vi "HelloWorld.vi"() -> ()   [LabVIEW 2018]
panel:
  out "error out":errorcluster
  in  "Name":string="World"
  out "response":string
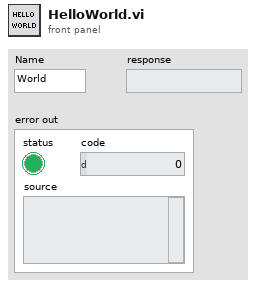
[diagram p1: front panel]
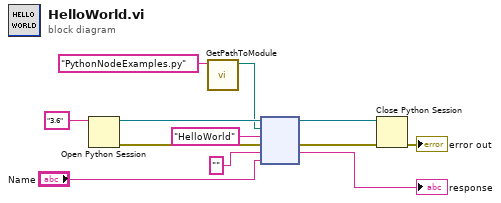
[diagram p0: block diagram]
diagram:
  n1 = Open Python Session(python version="3.6" ("Python version")) -> (session out=w12:refnum<k35>, error out=w4:errorcluster)  [unwired: 2 in]
  n2 = call "GetPathToModule.vi"("module name"="PythonNodeExamples.py") -> ("path to module"=w5:path)  [unwired: 10 in]
  n3 = node(w12, w5, "HelloWorld" ("function name"), w4, "", "Name") -> (w11:refnum<k35>, w3:errorcluster, →"response":string)  [unwired: 1 in, 2 out]
  n4 = Close Python Session(session in=w11, error in=w3) -> (11:→"error out":errorcluster)
